vi "ard_solucionC.vi"() -> ()   [LabVIEW 2020]
uses:
  <vilib>/Instr/_visa.llb/VISA Configure Serial Port (Instr).vi
panel:
  in  "string":string
  out "concatenated string 2":string
  in  "OK Button":bool
  in  "VISA resource name":refnum<visa-resource-name>
  in  "OK Button 2":bool
  in  "stop":bool
  out "concatenated string":string
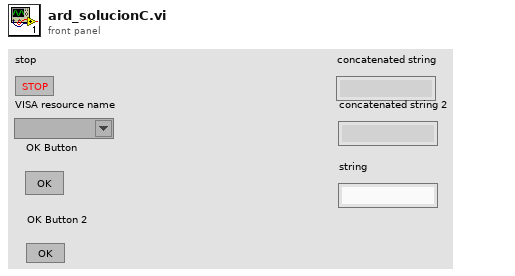
[diagram p1: front panel]
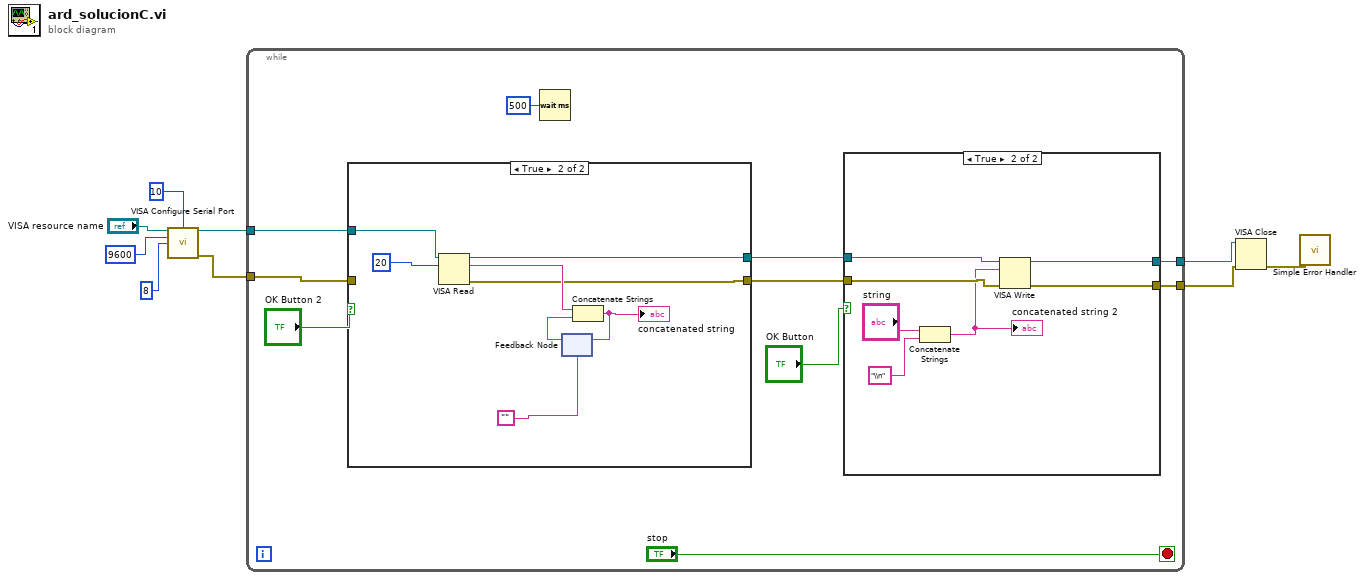
[diagram p0: block diagram]
diagram:
  n1 = call-poly "VISA Configure Serial Port"("VISA resource name"="VISA resource name", "termination char\n(0xA = '\\n' = LF)"=u8 10 ("termination char\n(0xA = '\\n' = LF)"), "baud rate (9600)"=u32 9600, "data bits (8)"=u16 8) -> ("VISA resource name out"=w9:refnum<visa-resource-name>, "error out"=w8:errorcluster)  [unwired: 10 in]
  n2 = while {
    tunnel: w9 -> [w18]
    tunnel: w8 -> [w17]
    tunnel: [w11] -> w3
    tunnel: [w10] -> w2
    stop <- "stop" stop-if-true
    n3 = case shown="True" "OK Button 2" {
      tunnel: [w29 w32] -> w14
      tunnel: [w30 w34] -> w13
      tunnel: w18 -> [w30 w33]
      tunnel: w17 -> [w29 _]
      frame False {
      }
      frame True {
        n4 = VISA Read(VISA resource name=w33, byte count=u32 20) -> (VISA resource name out=w34:refnum<visa-resource-name>, read buffer=w37:string, error out=w32:errorcluster)  [unwired: 1 in, 1 out]
        n5 = feedback #1("") -> (w35:string)
        n6 = Concatenate Strings(w37, w35) -> (w36:string)
        "concatenated string" <- w36
        n7 = feedback-in #1(w36) -> ()
      }
    }
    n8 = Wait (ms)(milliseconds to wait=u32 500) -> ()  [unwired: 1 out]
    n9 = case shown="True" "OK Button" {
      tunnel: w14 -> [w20 w27]
      tunnel: w13 -> [w21 w28]
      tunnel: [w21 w23] -> w11
      tunnel: [w20 w22] -> w10
      frame False {
      }
      frame True {
        n10 = Concatenate Strings("string", "\\n" ("string")) -> (w26:string)
        "concatenated string 2" <- w26
        n11 = VISA Write(VISA resource name=w28, write buffer=w26, error in (no error)=w27) -> (VISA resource name out=w23:refnum<visa-resource-name>, error out=w22:errorcluster)  [unwired: 1 out]
      }
    }
  }
  n12 = VISA Close(VISA resource name=w3, error in (no error)=w2) -> (error out=w1:errorcluster)
  n13 = call <vilib>:"Simple Error Handler.vi"("error in (no error)"=w1) -> ()  [unwired: 4 in, 5 out]
